vi "Timestamp to GPS Time.vi"(11 "Timestamp (now)":timestamp) -> (2 "Fractional Second":dbl, 3 "GPS Time (s)":i64)   [LabVIEW 2013]
uses:
  Epoch.GPS.lvclass
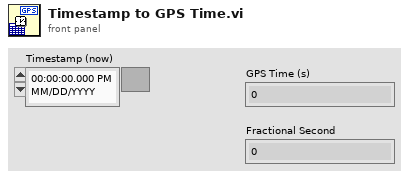
[diagram p1: front panel]
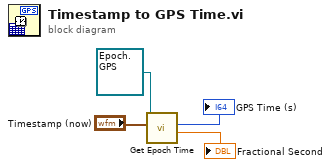
[diagram p0: block diagram]
diagram:
  n1 = call "Get Epoch Time.vi"("Timestamp (now)"="Timestamp (now)", "Epoch (Local)"=refnum<class "Epoch.GPS.lvclass"> refnum ("Epoch.GPS.lvclass")) -> ("Fractional Second"=→"Fractional Second":dbl, "Epoch Time (s)"=→"GPS Time (s)":i64)  [unwired: 7 in, 1 out]
